vi "LUCS001RT_GPS_GetLattitude.vi"(2 "LattitudeString":string) -> (5 "Lattitude.Degrees":i32, 7 "Lattitude.Minutes":dbl)   [LabVIEW 2020]
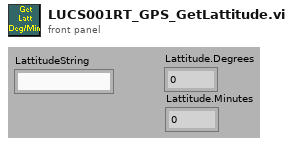
[diagram p1: front panel]
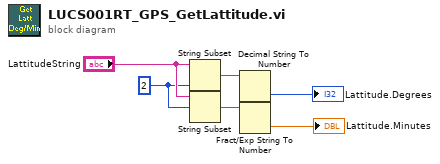
[diagram p0: block diagram]
diagram:
  w1 = 2 ("length (rest)")
  n1 = String Subset(string="LattitudeString", length (rest)=w1) -> (substring=w3:string)  [unwired: 1 in]
  n2 = String Subset(string="LattitudeString", offset (0)=w1) -> (substring=w4:string)  [unwired: 1 in]
  n3 = Decimal String To Number(string=w3) -> (number=→"Lattitude.Degrees":i32)  [unwired: 2 in, 1 out]
  n4 = Fract/Exp String To Number(string=w4) -> (number=→"Lattitude.Minutes":dbl)  [unwired: 3 in, 1 out]
